vi "TWO AXIS (Incremental Input).vi"() -> ()   [LabVIEW 2014]
uses:
  Control 1.ctl
  <vilib>/Instr/_visa.llb/VISA Flush IO Buffer Mask.ctl
  <vilib>/Instr/_visa.llb/VISA Configure Serial Port (Instr).vi
panel:
  in  "Mechanical Y Max":dbl
  in  "Mechanical X Max":dbl
  in  "X Min":dbl
  in  "Y Increment":dbl
  in  "Y Max":dbl
  in  "Y Min":dbl
  in  "X Increment":dbl
  in  "X Max":dbl
  in  "?":bool
  # "All Values are in cm."
  # "System operates by moving to a given Y-Value,\nthen iterates through all X values. After all Y-Values\nare complete the program waits for user confirmation\nthen returns to (0,0)."
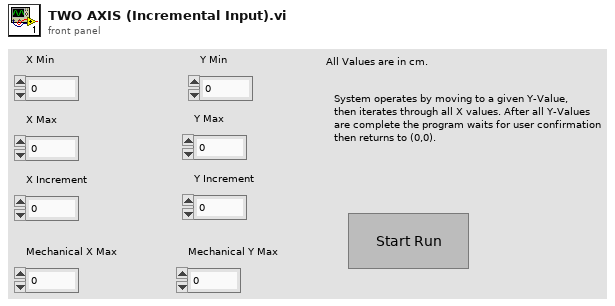
[diagram p1: front panel]
types:
  T1 = typedef "Control 1.ctl" = enum16{"Start", "Init", "Await Arduino Response", "Calculate Move", "Execute Move", "Home"}
  T2 = typedef "VISA Flush IO Buffer Mask.ctl" = u16
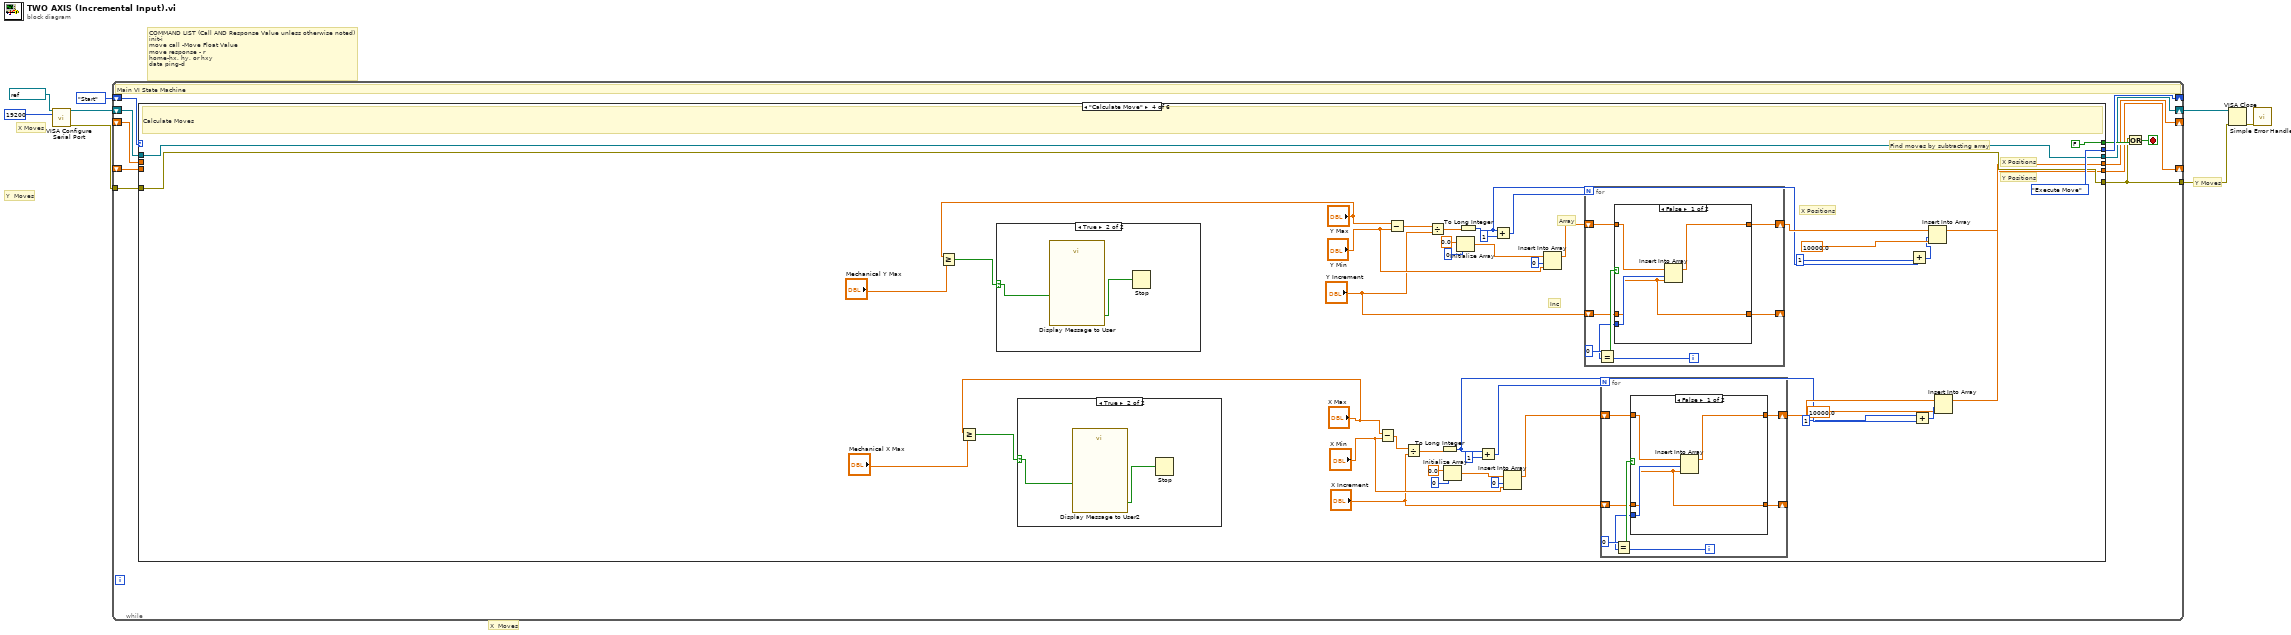
[diagram p0: block diagram]
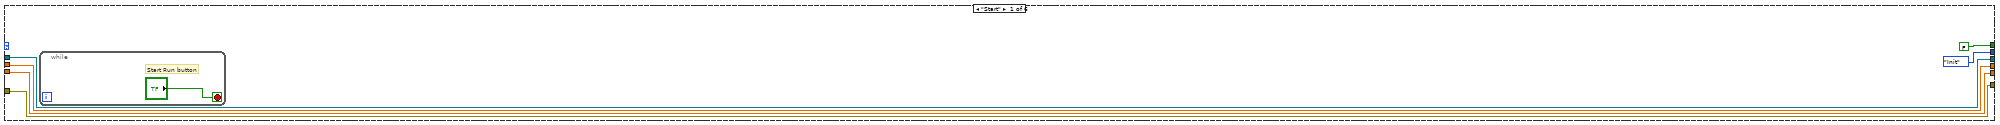
[diagram p2: hidden frame]
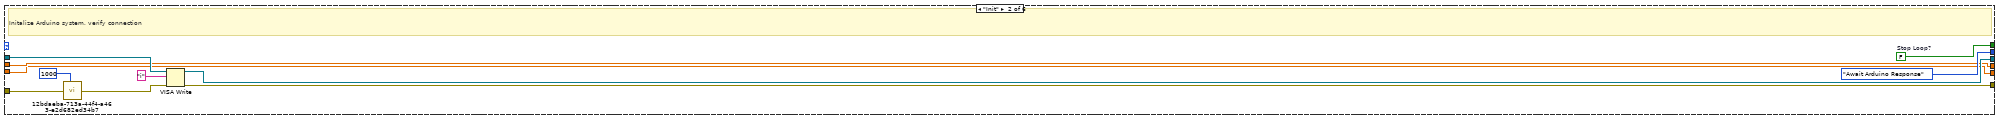
[diagram p3: hidden frame]
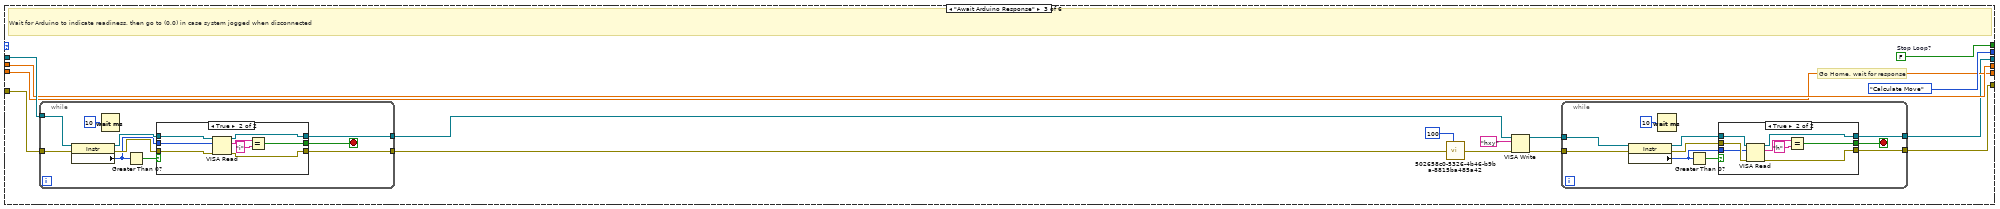
[diagram p4: hidden frame]
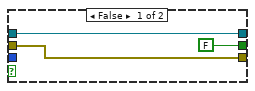
[diagram p5: hidden frame]
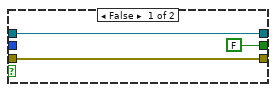
[diagram p6: hidden frame]
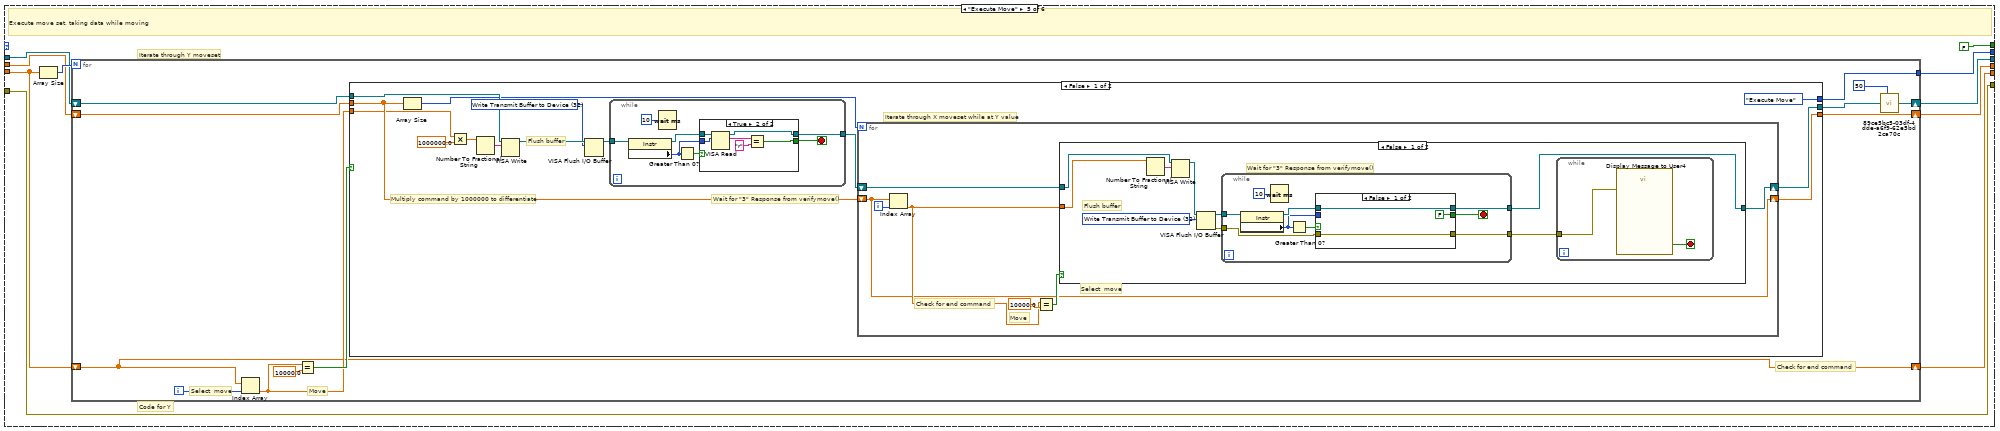
[diagram p11: hidden frame]
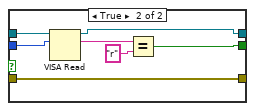
[diagram p12: hidden frame]
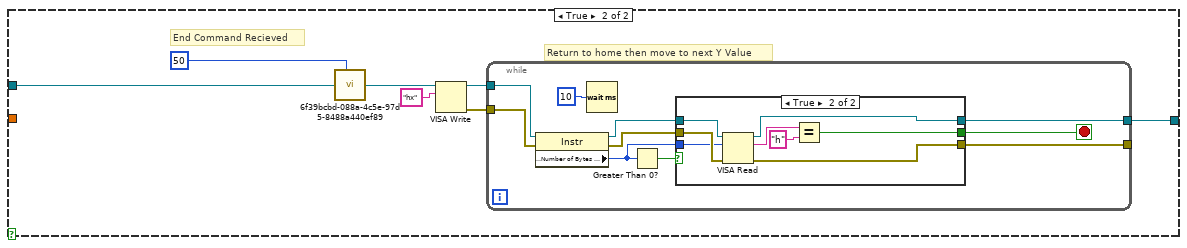
[diagram p13: hidden frame]
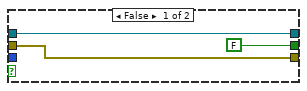
[diagram p14: hidden frame]
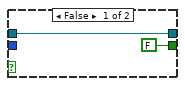
[diagram p15: hidden frame]
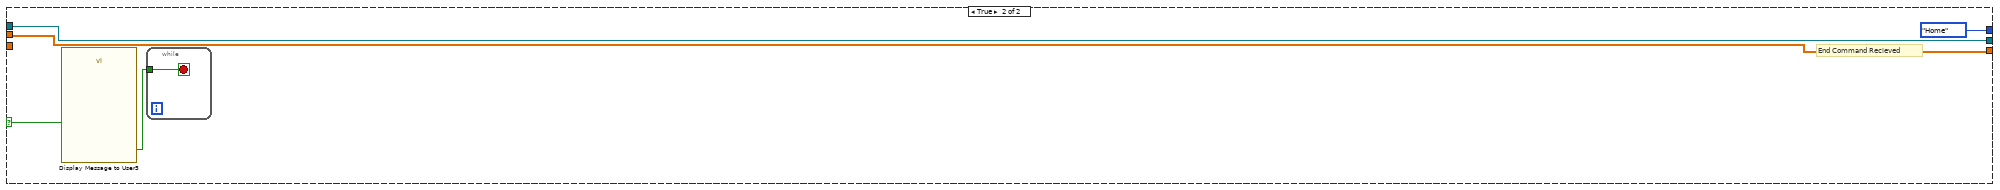
[diagram p16: hidden frame]
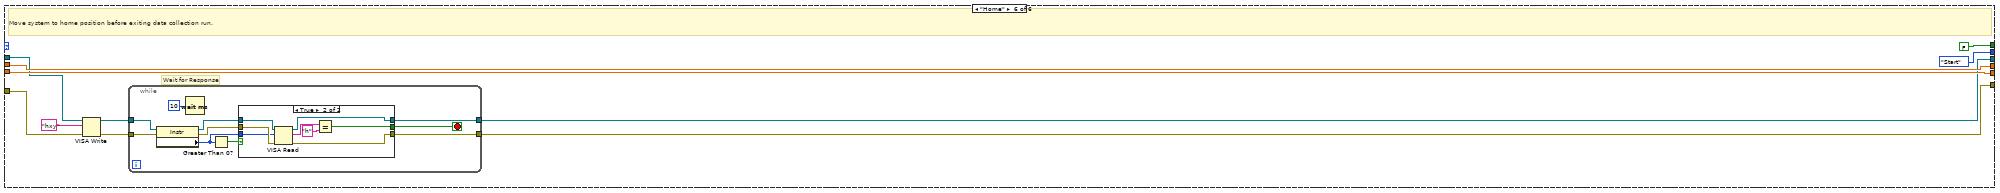
[diagram p17: hidden frame]
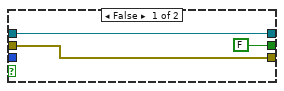
[diagram p18: hidden frame]
diagram:
  # "X  Moves"
  # "COMMAND LIST (Call AND Response Value unless otherwise noted)\ninit-i\nmove call -Move Float Value\nmove response - r\nhome-hx, hy, or hxy\ndata ping-d"
  # "Y Moves"
  # "X Moves"
  # "Y  Moves"
  n1 = call-poly "VISA Configure Serial Port"("VISA resource name"=refnum<visa-resource-name> "COM9", "baud rate (9600)"=u32 19200) -> ("VISA resource name out"=w6:refnum<visa-resource-name>, "error out"=w2:errorcluster)  [unwired: 12 in]
  n2 = while {
    shift-right: [w19] -> _
    shift-left: Control_1."Start" -> [w20]
    shift-right: [w16] -> w5
    shift-left: w6 -> [w17]
    shift-right: [w15] -> _
    shift-left: _ -> [w13]
    shift-right: [w14] -> _
    shift-left: _ -> [w12]
    tunnel: w2 -> [w11]
    tunnel: [w10] -> w1
    stop <- w9 stop-if-true
    # "Main VI State Machine"
    n3 = case shown="\"Calculate Move\"" w20 {
      tunnel: [Control_1."Init" Control_1."Await Arduino Response" Control_1."Calculate Move" Control_1."Execute Move" w173 Control_1."Start"] -> w19
      tunnel: [FALSE ("Stop Loop?") w38 w53 FALSE FALSE FALSE ("Stop Loop?")] -> w18
      tunnel: w17 -> [w23 w32 w52 w137 w170 w298]
      tunnel: w11 -> [w24 w34 w51 w136 w174 w297]
      tunnel: [w23 w35 w40 w137 w175 w293] -> w16
      tunnel: [w24 w36 w39 w136 w174 w292] -> w10
      tunnel: [w26 w29 w49 w103 w171 w300] -> w15
      tunnel: [w25 w28 w48 w102 w176 w299] -> w14
      tunnel: w13 -> [w26 w29 w49 _ w172 w300]
      tunnel: w12 -> [w25 w28 w48 _ w177 w299]
      frame "Start" {
        n4 = while {
          stop <- "?" stop-if-true
          # "Start Run button"
        }
      }
      frame "Init" {
        w38 = FALSE  # Stop Loop?
        # "Initalize Arduino system, verify connection"
        n5 = call "12bdaeba-713a-44f4-a463-e2d682ed34b7.vi"("value in"=w34, "milliseconds to wait"=u32 1000) -> ("value out"=w33:errorcluster)  [unwired: 1 out]
        n6 = VISA Write(VISA resource name=w32, write buffer="i", error in (no error)=w33) -> (VISA resource name out=w35:refnum<visa-resource-name>, error out=w36:errorcluster)  [unwired: 1 out]
      }
      frame "Await Arduino Response" {
        w53 = FALSE  # Stop Loop?
        # "Go Home, wait for response"
        # "Wait for Arduino to indicate readiness, then go to (0,0) in case system jogged when disconnected"
        n7 = while {
          tunnel: w52 -> [w84]
          tunnel: w51 -> [w83]
          tunnel: [w77] -> w42
          tunnel: [w76] -> w47
          stop <- w78 stop-if-true
          n8 = property class="Instr"(reference=w84, error in=w83) -> (reference out=w81:refnum<visa-resource-name>, error out=w80:errorcluster, "Serial Settings:Number of Bytes at Serial Port"=w79:u32)
          n9 = Wait (ms)(milliseconds to wait=u32 10) -> ()  [unwired: 1 out]
          n10 = Greater Than 0?(x=w79) -> (x > 0?=w82:bool)
          n11 = case shown="True" w82 {
            tunnel: w81 -> [w87 w95]
            tunnel: w80 -> [w86 w94]
            tunnel: w79 -> [_ w93]
            tunnel: [FALSE w89] -> w78
            tunnel: [w87 w91] -> w77
            tunnel: [w86 w90] -> w76
            frame False {
            }
            frame True {
              n12 = VISA Read(VISA resource name=w95, byte count=w93, error in (no error)=w94) -> (VISA resource name out=w91:refnum<visa-resource-name>, read buffer=w88:string, error out=w90:errorcluster)  [unwired: 1 out]
              n13 = Equal?(x=w88, y="i") -> (x = y?=w89:bool)
            }
          }
        }
        n14 = call "502658c0-5326-4b46-b9ba-8815ba485a42.vi"("value in"=w47, "milliseconds to wait"=u32 100) -> ("value out"=w41:errorcluster)  [unwired: 1 out]
        n15 = VISA Write(VISA resource name=w42, write buffer="hxy", error in (no error)=w41) -> (VISA resource name out=w44:refnum<visa-resource-name>, error out=w43:errorcluster)  [unwired: 1 out]
        n16 = while {
          tunnel: w44 -> [w63]
          tunnel: w43 -> [w62]
          tunnel: [w56] -> w40
          tunnel: [w55] -> w39
          stop <- w57 stop-if-true
          n17 = property class="Instr"(reference=w63, error in=w62) -> (reference out=w60:refnum<visa-resource-name>, error out=w59:errorcluster, "Serial Settings:Number of Bytes at Serial Port"=w58:u32)
          n18 = Wait (ms)(milliseconds to wait=u32 10) -> ()  [unwired: 1 out]
          n19 = Greater Than 0?(x=w58) -> (x > 0?=w61:bool)
          n20 = case shown="True" w61 {
            tunnel: w60 -> [w66 w74]
            tunnel: w59 -> [w65 w73]
            tunnel: w58 -> [_ w72]
            tunnel: [FALSE w68] -> w57
            tunnel: [w66 w70] -> w56
            tunnel: [w65 w69] -> w55
            frame False {
            }
            frame True {
              n21 = VISA Read(VISA resource name=w74, byte count=w72, error in (no error)=w73) -> (VISA resource name out=w70:refnum<visa-resource-name>, read buffer=w67:string, error out=w69:errorcluster)  [unwired: 1 out]
              n22 = Equal?(x=w67, y="h") -> (x = y?=w68:bool)
            }
          }
        }
      }
      frame "Calculate Move" {
        # "Inc"
        # "Array"
        # "X Positions"
        # "Find moves by subtracting array"
        # "X Positions"
        # "Y Positions"
        # "Calculate Moves"
        n23 = Greater Or Equal?(x="Y Max", y="Mechanical Y Max") -> (x >= y?=w100:bool)
        n24 = Greater Or Equal?(x="X Max", y="Mechanical X Max") -> (x >= y?=w99:bool)
        n25 = case shown="True" w100 {
          selector: w100 -> [_ w143]
          frame False {
          }
          frame True {
            n26 = call "Display Message to User"("Enable"=w143) -> ("OK"=w142:bool)  [unwired: 9 in, 1 out]
            n27 = Stop(stop? (T)=w142) -> ()
          }
        }
        n28 = case shown="True" w99 {
          selector: w99 -> [_ w140]
          frame False {
          }
          frame True {
            n29 = call "Display Message to User2"("Enable"=w140) -> ("OK"=w141:bool)  [unwired: 9 in, 1 out]
            n30 = Stop(stop? (T)=w141) -> ()
          }
        }
        n31 = Subtract(x="X Max", y="X Min") -> (x-y=w134:dbl)
        n32 = Subtract(x="Y Max", y="Y Min") -> (x-y=w135:dbl)
        n33 = Divide(x=w134, y="X Increment") -> (x/y=w133:dbl)
        n34 = Divide(x=w135, y="Y Increment") -> (x/y=w132:dbl)
        n35 = To Long Integer(number=w133) -> (32bit integer=w107:i32)
        n36 = Initialize Array(0.0 ("element"), 0 ("dimension size")) -> (w120:dbl[])
        n37 = Initialize Array(0.0 ("element"), 0 ("dimension size")) -> (w123:dbl[])
        n38 = To Long Integer(number=w132) -> (32bit integer=w111:i32)
        n39 = Add(x=w107, y=1) -> (x+y=w114:i32)
        n40 = Add(x=w111, y=1) -> (x+y=w117:i32)
        n41 = Insert Into Array(array=w120, index=0, new element="X Min") -> (w116:dbl[])
        n42 = Insert Into Array(array=w123, index=0, new element="Y Min") -> (w119:dbl[])
        n43 = for {
          N: w117 -> [_]
          shift-right: [w160] -> w113
          shift-left: w119 -> [w161]
          shift-right: [w158] -> _
          shift-left: "Y Increment" -> [w159]
          i -> [w157]
          n44 = Equal?(x=0, y=w157) -> (x = y?=w162:bool)
          n45 = case shown="False" w162 {
            tunnel: w161 -> [w166 w169]
            tunnel: [w165 w169] -> w160
            tunnel: w159 -> [w164 w168]
            tunnel: [w164 w168] -> w158
            tunnel: w157 -> [w167 _]
            frame False {
              n46 = Insert Into Array(array=w166, index=w167, new element=w164) -> (w165:dbl[])
            }
            frame True {
            }
          }
        }
        n47 = for {
          N: w114 -> [_]
          shift-right: [w147] -> w108
          shift-left: w116 -> [w148]
          shift-right: [w145] -> _
          shift-left: "X Increment" -> [w146]
          i -> [w144]
          n48 = Equal?(x=0, y=w144) -> (x = y?=w149:bool)
          n49 = case shown="False" w149 {
            tunnel: w148 -> [w153 w156]
            tunnel: [w152 w156] -> w147
            tunnel: w146 -> [w151 w155]
            tunnel: [w151 w155] -> w145
            tunnel: w144 -> [w154 _]
            frame False {
              n50 = Insert Into Array(array=w153, index=w154, new element=w151) -> (w152:dbl[])
            }
            frame True {
            }
          }
        }
        n51 = Add(x=1, y=w111) -> (x+y=w109:i32)
        n52 = Add(x=1, y=w107) -> (x+y=w105:i32)
        n53 = Insert Into Array(array=w113, index=w109, new element=10000.0 ("new element/subarray")) -> (w102:dbl[])
        n54 = Insert Into Array(array=w108, index=w105, new element=10000.0 ("new element/subarray")) -> (w103:dbl[])
      }
      frame "Execute Move" {
        # "Iterate through Y moveset"
        # "Code for Y"
        # "Execute move set, taking data while moving"
        n55 = Array Size(array=w177) -> (size(s)=w178:i32)
        n56 = for {
          N: w178 -> [_]
          shift-right: [w187] -> w176
          shift-left: w177 -> [w187]
          tunnel: [w186] -> w173
          shift-right: [w183] -> w175
          shift-left: w170 -> [w185]
          shift-right: [w180] -> w171
          shift-left: w172 -> [w181]
          i -> [w191]
          # "Select  move"
          # "Check for end command"
          # "Move"
          n57 = Index Array(array=w187, index=w191) -> (element=w188:dbl)
          n58 = Equal?(x=w188, y=10000.0) -> (x = y?=w189:bool)
          n59 = case shown="False" w189 {
            selector: w189 -> [_ w289]
            tunnel: w188 -> [w194 _]
            tunnel: [Control_1."Execute Move" Control_1."Home"] -> w186
            tunnel: w185 -> [w204 w287]
            tunnel: [w197 w287] -> w184
            tunnel: w181 -> [w196 w286]
            tunnel: [w198 w286] -> w180
            frame False {
              w200 = T2 32 items=["Flush Receive Buffer"=16, "Write Transmit Buffer to Device"=32, "Flush Receive Buffer (No I/O)"=64, "Flush Transmit Buffer"=128] ("Mask")
              # "Flush buffer"
              # "Iterate through X moveset while at Y value"
              # "Multiply command by 1000000 to differentiate"
              # "Wait for \"3\" Response from verifymove()"
              n60 = Array Size(array=w196) -> (size(s)=w195:i32)
              n61 = Multiply(x=w194, y=1000000.0) -> (x*y=w193:dbl)
              n62 = Number To Fractional String(number=w193) -> (F-format string=w203:string)  [unwired: 3 in]
              n63 = VISA Write(VISA resource name=w204, write buffer=w203) -> (VISA resource name out=w202:refnum<visa-resource-name>)  [unwired: 1 in, 2 out]
              n64 = VISA Flush I/O Buffer(VISA resource name=w202, mask (16)=w200) -> (VISA resource name out=w201:refnum<visa-resource-name>)  [unwired: 1 in, 1 out]
              n65 = while {
                tunnel: w201 -> [w277]
                tunnel: [w272] -> w199
                stop <- w273 stop-if-true
                n66 = property class="Instr"(reference=w277) -> (reference out=w275:refnum<visa-resource-name>, "Serial Settings:Number of Bytes at Serial Port"=w274:u32)  [unwired: 1 in, 1 out]
                n67 = Wait (ms)(milliseconds to wait=u32 10) -> ()  [unwired: 1 out]
                n68 = Greater Than 0?(x=w274) -> (x > 0?=w276:bool)
                n69 = case shown="True" w276 {
                  tunnel: w275 -> [w279 w285]
                  tunnel: w274 -> [_ w284]
                  tunnel: [FALSE w282] -> w273
                  tunnel: [w279 w283] -> w272
                  frame False {
                  }
                  frame True {
                    n70 = VISA Read(VISA resource name=w285, byte count=w284) -> (VISA resource name out=w283:refnum<visa-resource-name>, read buffer=w281:string)  [unwired: 1 in, 2 out]
                    n71 = Equal?(x=w281, y="r") -> (x = y?=w282:bool)
                  }
                }
              }
              n72 = for {
                N: w195 -> [_]
                shift-right: [w207] -> w198
                shift-left: w196 -> [w207]
                shift-right: [w206] -> w197
                shift-left: w199 -> [w208]
                i -> [w212]
                # "Check for end command"
                # "Move"
                # "Select  move"
                n73 = Index Array(array=w207, index=w212) -> (element=w209:dbl)
                n74 = Equal?(x=w209, y=10000.0) -> (x = y?=w210:bool)
                n75 = case shown="False" w210 {
                  tunnel: w209 -> [w220 _]
                  tunnel: w208 -> [w221 w245]
                  tunnel: [w214 w246] -> w206
                  frame False {
                    w216 = T2 32 items=["Flush Receive Buffer"=16, "Write Transmit Buffer to Device"=32, "Flush Receive Buffer (No I/O)"=64, "Flush Transmit Buffer"=128] ("Mask")
                    # "Flush buffer"
                    # "Wait for \"3\" Response from verifymove()"
                    n76 = Number To Fractional String(number=w220) -> (F-format string=w219:string)  [unwired: 3 in]
                    n77 = VISA Write(VISA resource name=w221, write buffer=w219) -> (VISA resource name out=w218:refnum<visa-resource-name>)  [unwired: 1 in, 2 out]
                    n78 = VISA Flush I/O Buffer(VISA resource name=w218, mask (16)=w216) -> (VISA resource name out=w217:refnum<visa-resource-name>, error out=w215:errorcluster)  [unwired: 1 in]
                    n79 = while {
                      tunnel: w217 -> [w232]
                      tunnel: [w227] -> w214
                      tunnel: w215 -> [w225]
                      tunnel: [w224] -> w213
                      stop <- w228 stop-if-true
                      n80 = property class="Instr"(reference=w232) -> (reference out=w230:refnum<visa-resource-name>, "Serial Settings:Number of Bytes at Serial Port"=w229:u32)  [unwired: 1 in, 1 out]
                      n81 = Wait (ms)(milliseconds to wait=u32 10) -> ()  [unwired: 1 out]
                      n82 = Greater Than 0?(x=w229) -> (x > 0?=w231:bool)
                      n83 = case shown="False" w231 {
                        tunnel: w230 -> [w235 w242]
                        tunnel: w229 -> [_ w241]
                        tunnel: [FALSE w239] -> w228
                        tunnel: [w235 w240] -> w227
                        tunnel: w225 -> [w233 w236]
                        tunnel: [w233 w236] -> w224
                        frame False {
                        }
                        frame True {
                          n84 = VISA Read(VISA resource name=w242, byte count=w241) -> (VISA resource name out=w240:refnum<visa-resource-name>, read buffer=w238:string)  [unwired: 1 in, 2 out]
                          n85 = Equal?(x=w238, y="r") -> (x = y?=w239:bool)
                        }
                      }
                    }
                    n86 = while {
                      tunnel: w213 -> [w223]
                      stop <- w222 stop-if-true
                      n87 = call "Display Message to User4"("error in (no error)"=w223) -> ("Continue"=w222:bool)  [unwired: 9 in, 1 out]
                    }
                  }
                  frame True {
                    # "Return to home then move to next Y Value"
                    # "End Command Recieved"
                    n88 = call "6f39bcbd-088a-4c5e-97d5-8488a440ef89.vi"("value in"=w245, "milliseconds to wait"=u32 50) -> ("value out"=w244:refnum<visa-resource-name>)  [unwired: 1 out]
                    n89 = VISA Write(VISA resource name=w244, write buffer="hx") -> (VISA resource name out=w248:refnum<visa-resource-name>, error out=w247:errorcluster)  [unwired: 1 in, 1 out]
                    n90 = while {
                      tunnel: w248 -> [w259]
                      tunnel: w247 -> [w258]
                      tunnel: [w252] -> w246
                      tunnel: [w251] -> _
                      stop <- w253 stop-if-true
                      n91 = property class="Instr"(reference=w259, error in=w258) -> (reference out=w256:refnum<visa-resource-name>, error out=w255:errorcluster, "Serial Settings:Number of Bytes at Serial Port"=w254:u32)
                      n92 = Wait (ms)(milliseconds to wait=u32 10) -> ()  [unwired: 1 out]
                      n93 = Greater Than 0?(x=w254) -> (x > 0?=w257:bool)
                      n94 = case shown="True" w257 {
                        tunnel: w256 -> [w262 w270]
                        tunnel: w255 -> [w261 w269]
                        tunnel: w254 -> [_ w268]
                        tunnel: [FALSE w264] -> w253
                        tunnel: [w262 w266] -> w252
                        tunnel: [w261 w265] -> w251
                        frame False {
                        }
                        frame True {
                          n95 = VISA Read(VISA resource name=w270, byte count=w268, error in (no error)=w269) -> (VISA resource name out=w266:refnum<visa-resource-name>, read buffer=w263:string, error out=w265:errorcluster)  [unwired: 1 out]
                          n96 = Equal?(x=w263, y="h") -> (x = y?=w264:bool)
                        }
                      }
                    }
                  }
                }
              }
            }
            frame True {
              # "End Command Recieved"
              n97 = call "Display Message to User3"("Enable"=w289) -> ("Return to Home"=w290:bool)  [unwired: 9 in, 1 out]
              n98 = while {
                tunnel: w290 -> [w291]
                stop <- w291 stop-if-true
              }
            }
          }
          n99 = call "89ce5bc5-03df-4dde-a6f9-62e5bd2ca70c.vi"("value in"=w184, "milliseconds to wait"=u32 50) -> ("value out"=w183:refnum<visa-resource-name>)  [unwired: 1 out]
        }
      }
      frame "Home" {
        # "Wait for Response"
        # "Move system to home position before exiting data collection run."
        n100 = VISA Write(VISA resource name=w298, write buffer="hxy", error in (no error)=w297) -> (VISA resource name out=w295:refnum<visa-resource-name>, error out=w294:errorcluster)  [unwired: 1 out]
        n101 = while {
          tunnel: w295 -> [w312]
          tunnel: w294 -> [w311]
          tunnel: [w305] -> w293
          tunnel: [w304] -> w292
          stop <- w306 stop-if-true
          n102 = property class="Instr"(reference=w312, error in=w311) -> (reference out=w309:refnum<visa-resource-name>, error out=w308:errorcluster, "Serial Settings:Number of Bytes at Serial Port"=w307:u32)
          n103 = Wait (ms)(milliseconds to wait=u32 10) -> ()  [unwired: 1 out]
          n104 = Greater Than 0?(x=w307) -> (x > 0?=w310:bool)
          n105 = case shown="True" w310 {
            tunnel: w309 -> [w315 w323]
            tunnel: w308 -> [w314 w322]
            tunnel: w307 -> [_ w321]
            tunnel: [FALSE w317] -> w306
            tunnel: [w315 w319] -> w305
            tunnel: [w314 w318] -> w304
            frame False {
            }
            frame True {
              n106 = VISA Read(VISA resource name=w323, byte count=w321, error in (no error)=w322) -> (VISA resource name out=w319:refnum<visa-resource-name>, read buffer=w316:string, error out=w318:errorcluster)  [unwired: 1 out]
              n107 = Equal?(x=w316, y="h") -> (x = y?=w317:bool)
            }
          }
        }
      }
    }
    n108 = Or(x=w10, y=w18) -> (x .or. y?=w9:bool)
  }
  n109 = VISA Close(VISA resource name=w5, error in (no error)=w1) -> (error out=w7:errorcluster)
  n110 = call <vilib>:"Simple Error Handler.vi"("error in (no error)"=w7) -> ()  [unwired: 4 in, 5 out]
